vi "FileExcelOpen.vi"(6 "提示语":refnum<vi>, 7 "Language":u32, 8 "进度条":refnum<vi>, 9 "进度数值":refnum<vi>, 10 "报文行数统计":refnum<vi>, 11 "file path (dialog if empty)":path caption="文件路径 （空时为对话框）") -> (0 "路径输出":path, 1 "重构的Data数组":u32[][](array[numeric]), 2 "统计数量":string[](array[string]), 3 "报文ID":string[](array[string]), 4 "基时间簇":T1, 5 "CAN报文统计":string[][](array[string]))   [LabVIEW 2015]
uses:
  <vilib>/addons/_office/excel.llb/Excel Get Data ([str]).vi
  <vilib>/Utility/NIReport.llb/NI_report.lvclass
  <vilib>/addons/_office/NI_ReportGenerationToolkit.lvlib
  <vilib>/Utility/NIReport.llb/Excel/NI_Excel.lvclass
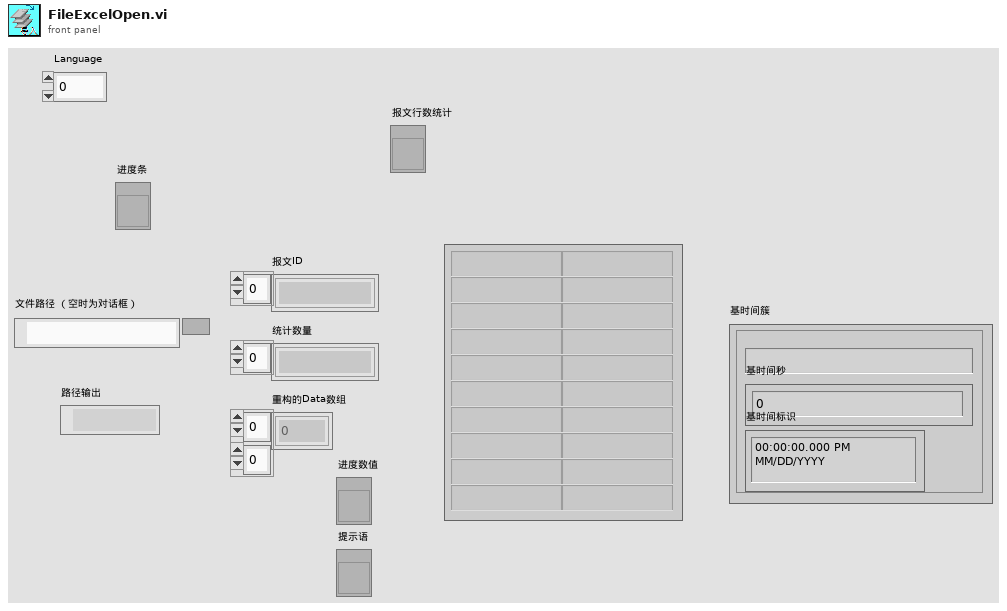
[diagram p1: front panel]
types:
  T1 = cluster{"基时间字符串":string, "基时间秒":dbl, "基时间标识":timestamp}
  T2 = enum16{"maximized", "minimized", "normal", "no change"}
  T3 = enum16{"Standard Report", "HTML", "Word", "Excel"}
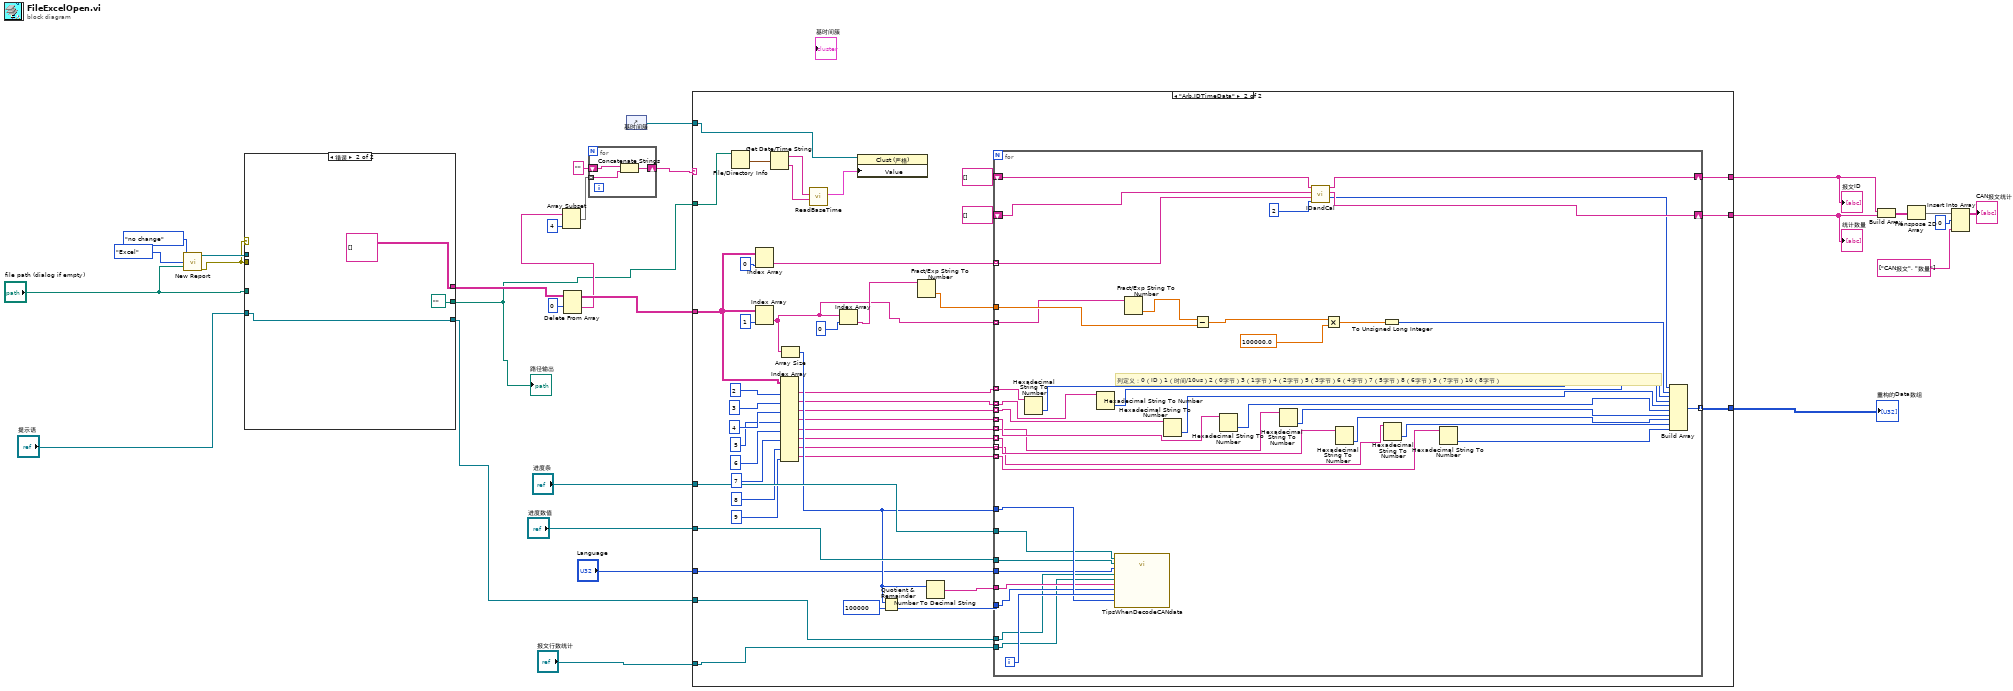
[diagram p0: block diagram]
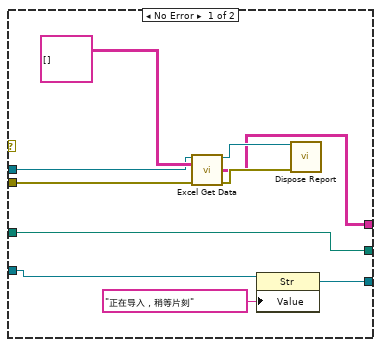
[diagram p2: hidden frame]
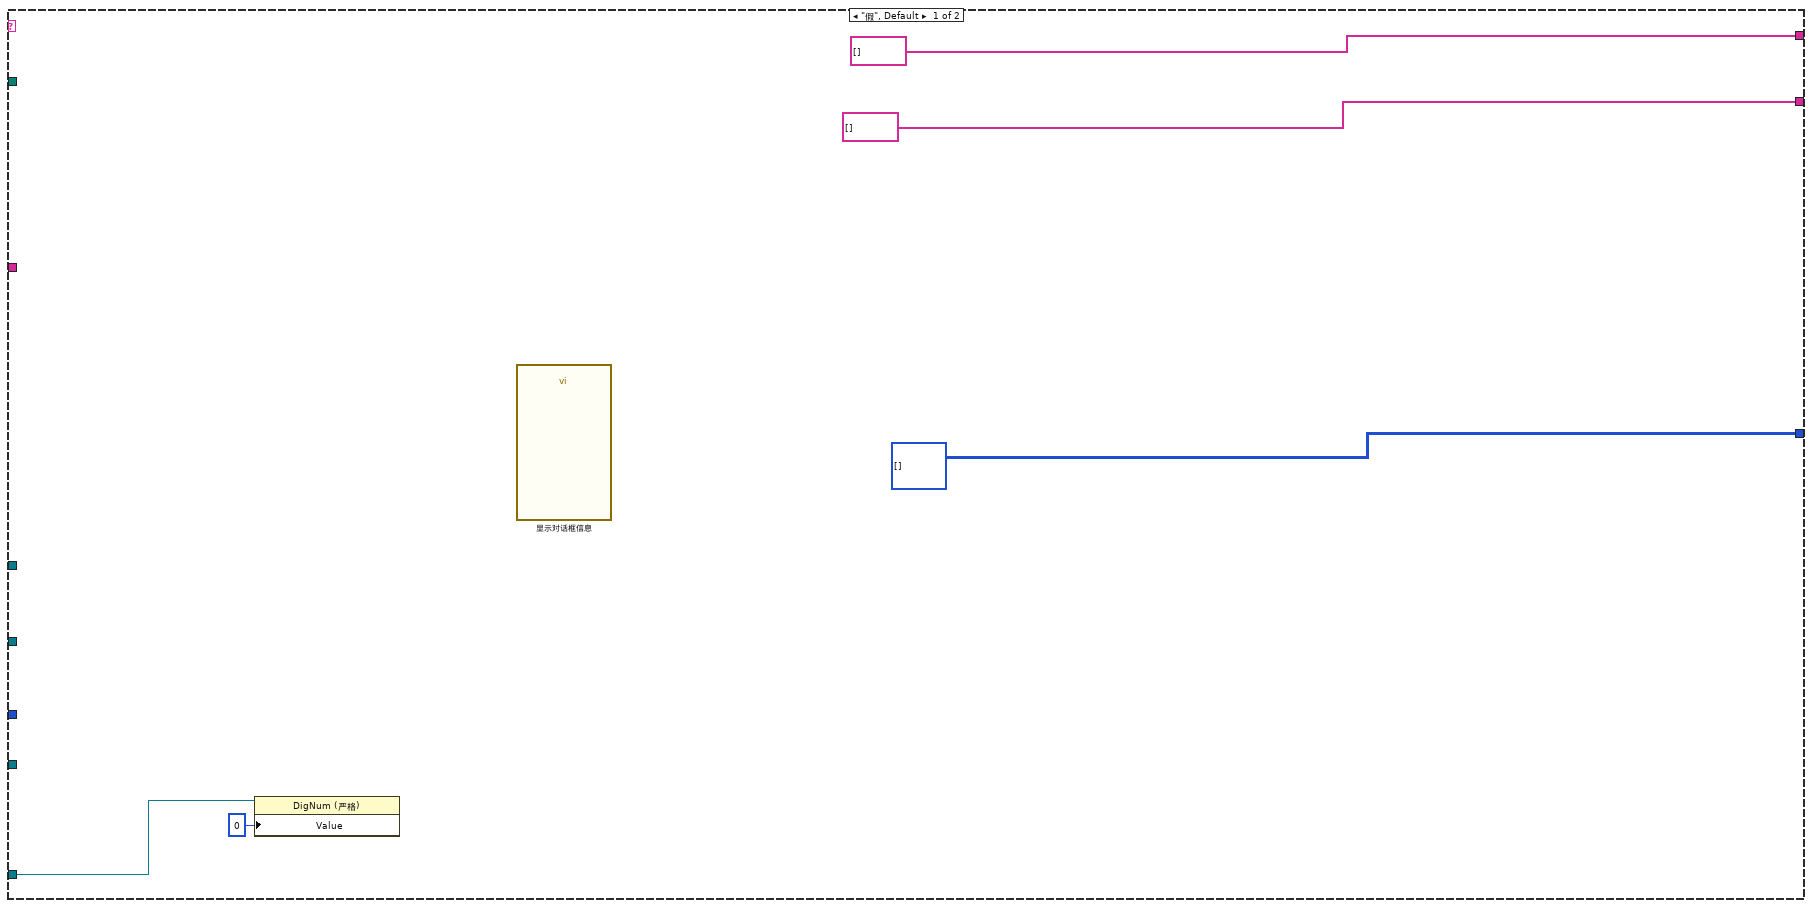
[diagram p3: hidden frame]
diagram:
  n1 = call <vilib>:"New Report.vi"("window state (normal)"=T2."no change", "report type"=T3."Excel", "template (empty)"="file path (dialog if empty)") -> ("report out"=w9:refnum<class "NI_report.lvclass">, "error out"=w5:errorcluster)  [unwired: 11 in]
  n2 = case shown="错误" w5 {
    tunnel: w9 -> [w38 _]
    tunnel: w5 -> [w37 _]
    tunnel: [w34 string[][] []] -> w6
    tunnel: "提示语" -> [w33 w41]
    tunnel: [w32 w41] -> w3
    tunnel: "file path (dialog if empty)" -> [w31 _]
    tunnel: [w31 path "" ("file path (dialog if empty)")] -> w1
    frame No Error {
      n3 = call-poly <vilib>:"Excel Get Data.vi"("report in"=w38, "data type"=string[][] [], "error in (no error)"=w37) -> ("report out"=w35:refnum<class "NI_report.lvclass">, "data"=w34:string[][], "error out"=w36:errorcluster)  [unwired: 10 in]
      n4 = property class="Str"(reference=w33, "Value"="正在导入，稍等片刻" ("值")) -> (reference out=w32:refnum<vi>)  [unwired: 1 in, 1 out]
      n5 = call-dynamic "Dispose Report.vi"("report in"=w35, "error in (no error)"=w36) -> ()  [unwired: 13 in, 1 out]
    }
    frame Error {
    }
  }
  "路径输出" <- w1
  n6 = Delete From Array(array=w6, index (row)=0 ("索引 (行)")) -> (deleted portion=w12:string[], array with subset deleted=w28:string[][])  [unwired: 2 in]
  n7 = Array Subset(array=w12, length=4 ("长度")) -> (w13:string[])  [unwired: 1 in]
  n8 = for {
    tunnel: w13 -> [w44] mode=indexing
    shift-right: [w45] -> w15
    shift-left: "" -> [w43]
    n9 = Concatenate Strings(w43, w44) -> (w45:string)
  }
  n10 = control-ref of="基时间簇"() -> (w11:refnum<vi>)
  n11 = case shown="\"Arb.IDTimeData\"" w15 {
    tunnel: [u32[][] [] w94] -> w29
    tunnel: w28 -> [_ w61]
    tunnel: [string[] [] w88] -> w22
    tunnel: [string[] [] w87] -> w21
    tunnel: "进度条" -> [_ w86]
    tunnel: "进度数值" -> [_ w85]
    tunnel: w3 -> [_ w82]
    tunnel: "报文行数统计" -> [w47 w74]
    tunnel: w11 -> [_ w76]
    tunnel: w1 -> [_ w78]
    tunnel: "Language" -> [_ w51]
    frame "假", Default {
      n12 = property class="DigNum (严格)"(reference=w47, "Value"=0 ("值")) -> ()  [unwired: 1 in, 2 out]
      n13 = call "显示对话框信息"() -> ()  [unwired: 10 in, 2 out]
    }
    frame "Arb.IDTimeData" {
      n14 = File/Directory Info(path=w78) -> (last mod=w79:timestamp)  [unwired: 1 in, 6 out]
      n15 = Index Array(array=w61, index (col)=0 ("禁用的索引 (列)")) -> (element=w93:string[])  [unwired: 1 in]
      n16 = Index Array(array=w61, index (col)=1 ("禁用的索引 (列)")) -> (element=w69:string[])  [unwired: 1 in]
      n17 = Get Date/Time String(seconds (now)=w79) -> (date string=w77:string, time string=w73:string)  [unwired: 2 in]
      n18 = Index Array(array=w61, index (col) #1=2 ("禁用的索引 (列)"), index (col) #2=3 ("禁用的索引 (列)"), index (col) #3=4 ("禁用的索引 (列)"), index (col) #4=5 ("禁用的索引 (列)"), index (col) #5=6 ("禁用的索引 (列)"), index (col) #6=7 ("禁用的索引 (列)"), index (col) #7=8 ("禁用的索引 (列)"), index (col) #8=9 ("禁用的索引 (列)")) -> (element #1=w60:string[], element #2=w58:string[], element #3=w57:string[], element #4=w56:string[], element #5=w55:string[], element #6=w54:string[], element #7=w53:string[], element #8=w52:string[])  [unwired: 8 in]
      n19 = Array Size(array=w69) -> (size(s)=w80:i32)
      n20 = call "ReadBaseTime.vi"("时间字符"=w73, "日期字符"=w77) -> ("基时间簇"=w75:T1)  [unwired: 7 in]
      n21 = Index Array(array=w69, index=0 ("索引")) -> (element=w71:string)
      n22 = property class="Clust (严格)"(reference=w76, "Value"=w75) -> ()  [unwired: 1 in, 2 out]
      n23 = Quotient & Remainder(x=w80, y=100000) -> (floor(x/y)=w83:i32)  [unwired: 1 out]
      n24 = Fract/Exp String To Number(string=w71) -> (number=w70:dbl)  [unwired: 3 in, 1 out]
      n25 = Number To Decimal String(number=w80) -> (decimal integer string=w81:string)  [unwired: 1 in]
      n26 = for {
        tunnel: w60 -> [w122] mode=indexing
        tunnel: [w126] -> w94 mode=indexing
        shift-right: [w101] -> w88
        shift-left: string[] [] -> [w95]
        shift-right: [w100] -> w87
        shift-left: string[] [] -> [w96]
        tunnel: w93 -> [w97] mode=indexing
        tunnel: w80 -> [w109]
        tunnel: w86 -> [w102]
        tunnel: w85 -> [w103]
        tunnel: w83 -> [w108]
        tunnel: w82 -> [w105]
        tunnel: w81 -> [w107]
        tunnel: w74 -> [w106]
        tunnel: w70 -> [w120]
        tunnel: w69 -> [w119] mode=indexing
        tunnel: w58 -> [w117] mode=indexing
        tunnel: w57 -> [w116] mode=indexing
        tunnel: w56 -> [w115] mode=indexing
        tunnel: w55 -> [w114] mode=indexing
        tunnel: w54 -> [w113] mode=indexing
        tunnel: w53 -> [w112] mode=indexing
        tunnel: w52 -> [w111] mode=indexing
        tunnel: w51 -> [w104]
        i -> [w110]
        # "列定义：0（ID）1（时间/10us）2（0字节）3（1字节）4（2字节）5（3字节）6（4字节）7（5字节）8（6字节）9（7字节）10（8字节）"
        n27 = Hexadecimal String To Number(string=w122) -> (number=w134:u32)  [unwired: 2 in, 1 out]
        n28 = Hexadecimal String To Number(string=w117) -> (number=w133:u32)  [unwired: 2 in, 1 out]
        n29 = call "TipsWhenDecodeCANdata.vi"("ProgressBar"=w102, "AllRowsNum"=w109, "i"=w110, "ProgressNum"=w103, "Language"=w104, "Tips"=w105, "MessageLinCnt"=w106, "txtAllRowsNum"=w107, "RowsLevel"=w108) -> ()  [unwired: 7 in]
        n30 = Fract/Exp String To Number(string=w119) -> (number=w121:dbl)  [unwired: 3 in, 1 out]
        n31 = Hexadecimal String To Number(string=w116) -> (number=w132:u32)  [unwired: 2 in, 1 out]
        n32 = Subtract(x=w121, y=w120) -> (x-y=w118:dbl)
        n33 = Hexadecimal String To Number(string=w115) -> (number=w131:u32)  [unwired: 2 in, 1 out]
        n34 = Hexadecimal String To Number(string=w114) -> (number=w130:u32)  [unwired: 2 in, 1 out]
        n35 = call "IDandCal.vi"("ID列表In"=w95, "数量统计in"=w96, "ID输入"=w97, "偏移量(0)"=2) -> ("ID列表"=w101:string[], "数量统计"=w100:string[], "ID输出"=w99:u32)  [unwired: 3 in]
        n36 = Multiply(x=w118, y=100000.0) -> (x*y=w124:dbl)
        n37 = Hexadecimal String To Number(string=w113) -> (number=w129:u32)  [unwired: 2 in, 1 out]
        n38 = To Unsigned Long Integer(number=w124) -> (unsigned 32bit integer=w123:u32)
        n39 = Hexadecimal String To Number(string=w112) -> (number=w128:u32)  [unwired: 2 in, 1 out]
        n40 = Hexadecimal String To Number(string=w111) -> (number=w127:u32)  [unwired: 2 in, 1 out]
        n41 = Build Array(w99, w123, w134, w133, w132, w131, w130, w129, w128, w127) -> (w126:u32[])
      }
    }
  }
  "重构的Data数组" <- w29
  "报文ID" <- w22
  "统计数量" <- w21
  n42 = Build Array(w22, w21) -> (w26:string[][])
  n43 = Transpose 2D Array(2D array=w26) -> (transposed array=w25:string[][])
  n44 = Insert Into Array(array=w25, index (row)=0 ("索引 (行)"), new element=string[] ["CAN报文", "数量"]) -> (→"CAN报文统计":string[][])  [unwired: 1 in]
